vi "Save File Create Default Configuration File.vi"(6 "delimiter (\\t)":string=",", 7 "Default File Create":T1, 8 "Error In":errorcluster={"status"=TRUE, "code"=1172, "source"="Invoke Node System.Reflection.TargetInvocationException: Exception has been thrown by the target of an invocation.\n\tInner Exception: System.ArgumentOutOfRangeException: Index was out of range. Must be non-negative and less than the size of the collection.\r\nParameter name: index <append><b>System.ArgumentOutOfRangeException</b> in GEA2_Toolkit.lvlib:GEA2 Initialize.vi->UTILITY Read Config File.vi->UTILITY Startup and Initialize.vi->HEWH RLT PRAT.vi"}, 11 "File Path In":path=path "C:/Work/Newfi Configuration_StationA.ini") -> (0 "Error Out":errorcluster={"status"=TRUE, "code"=1172, "source"="Invoke Node System.Reflection.TargetInvocationException: Exception has been thrown by the target of an invocation.\n\tInner Exception: System.ArgumentOutOfRangeException: Index was out of range. Must be non-negative and less than the size of the collection.\r\nParameter name: index <append><b>System.ArgumentOutOfRangeException</b> in GEA2_Toolkit.lvlib:GEA2 Initialize.vi->UTILITY Read Config File.vi->UTILITY Startup and Initialize.vi->HEWH RLT PRAT.vi"}, 3 "File Path Out":path=path "C:/Work/Newfi Configuration_StationA_StationD.ini")   [LabVIEW 2020]
uses:
  Type Definitions/UTILITY Default File Create.ctl
  <vilib>/Utility/file.llb/Write Delimited Spreadsheet (string).vi
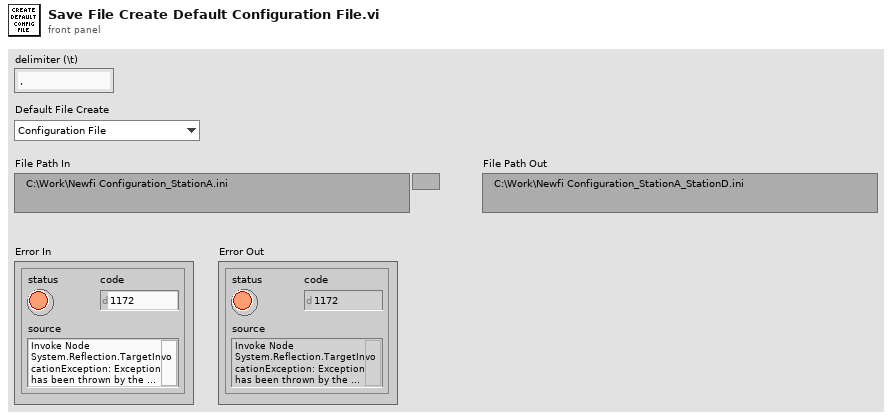
[diagram p1: front panel]
types:
  T1 = typedef "UTILITY Default File Create.ctl" = enum16{"Configuration File", "Debug Search File", "WILT Water Injection Times", "WILT Agilent Assignment", "WILT Save Status Path", "WILT General Config"}
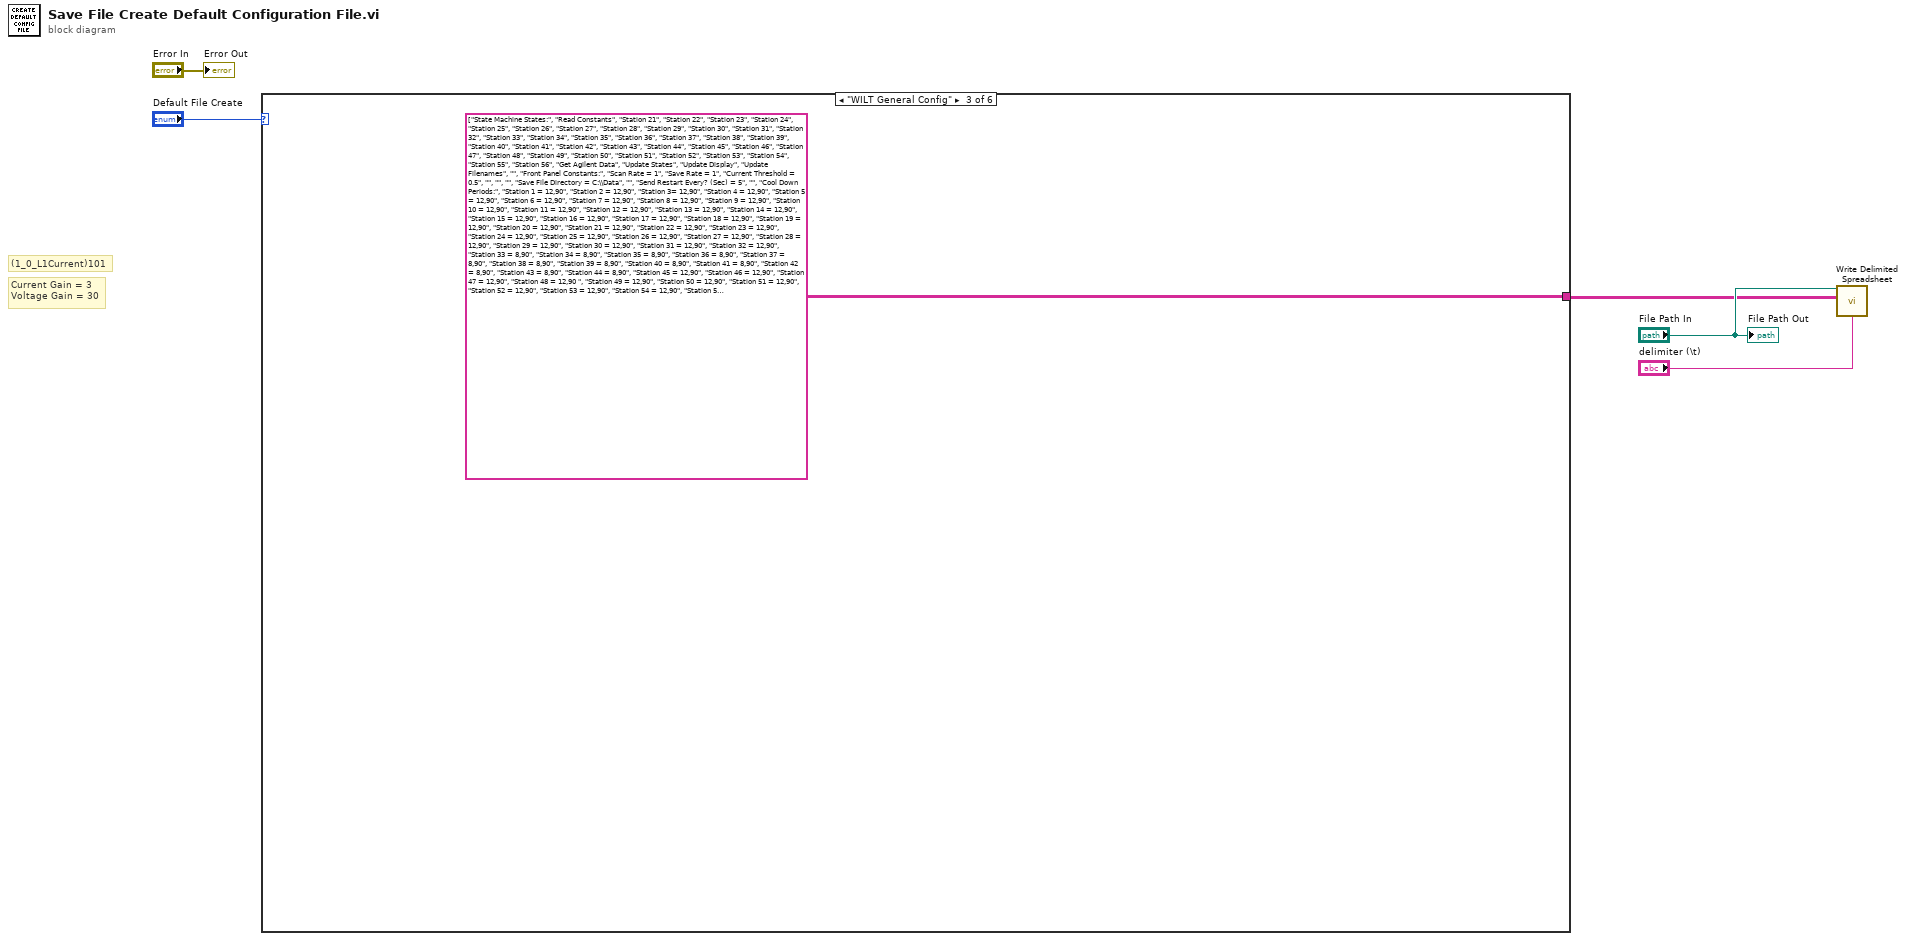
[diagram p0: block diagram]
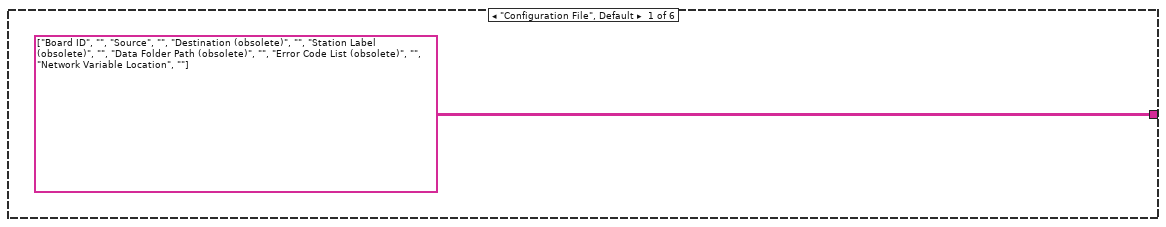
[diagram p2: hidden frame]
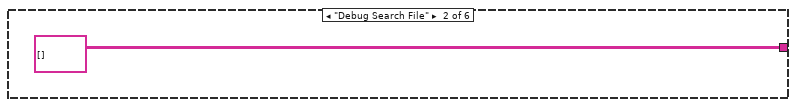
[diagram p3: hidden frame]
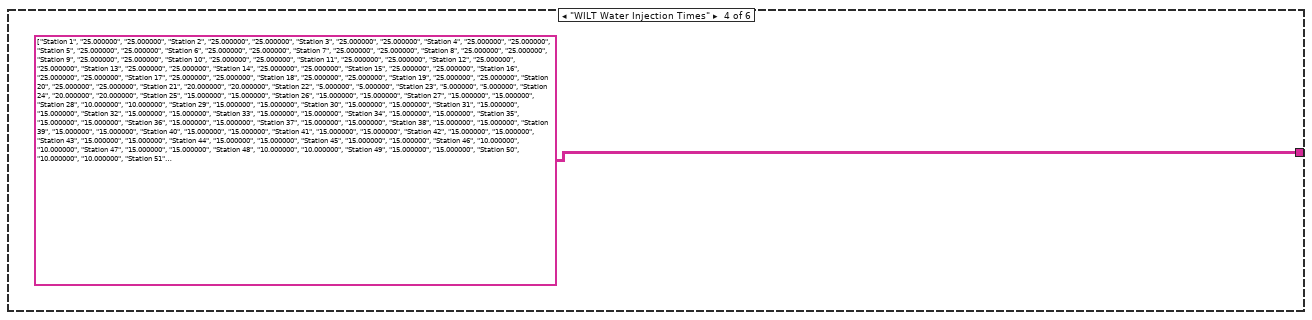
[diagram p4: hidden frame]
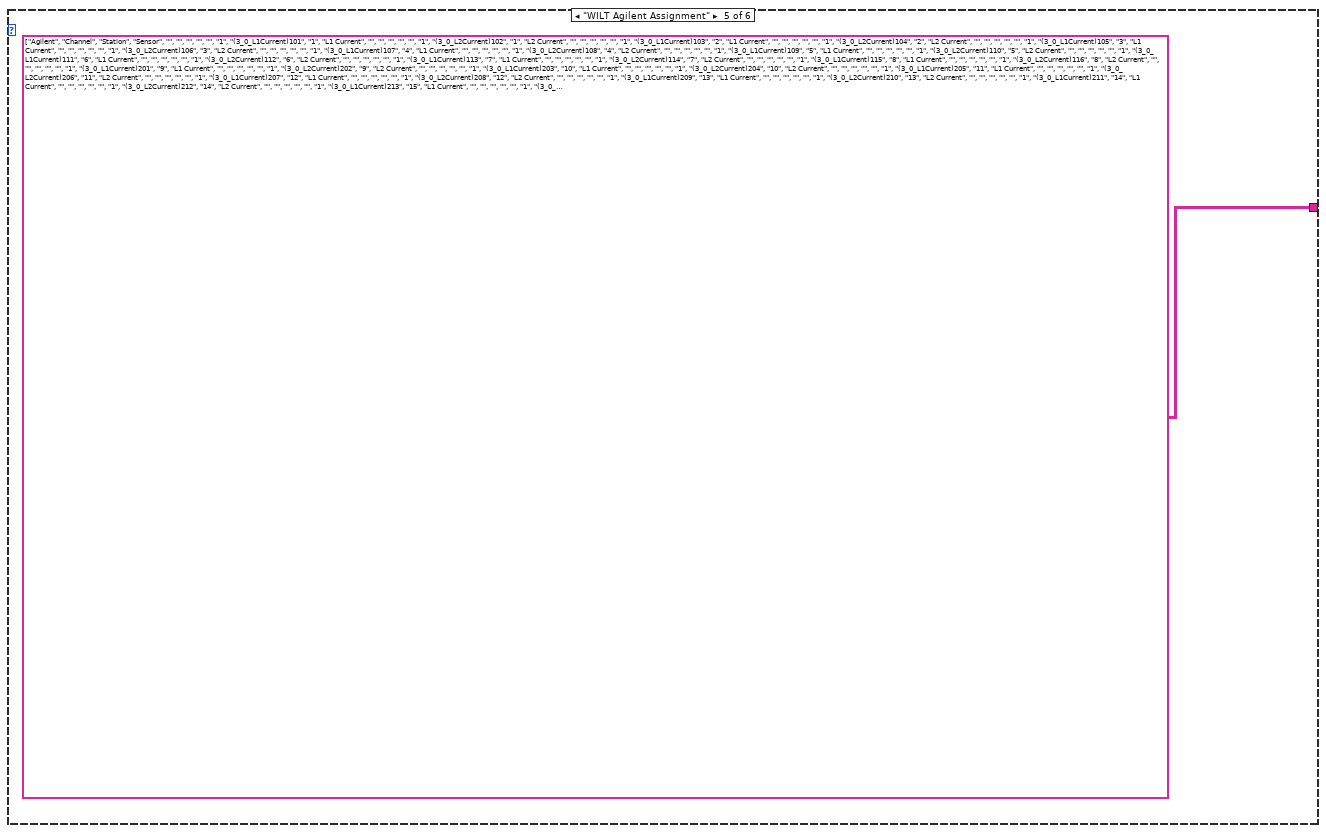
[diagram p5: hidden frame]
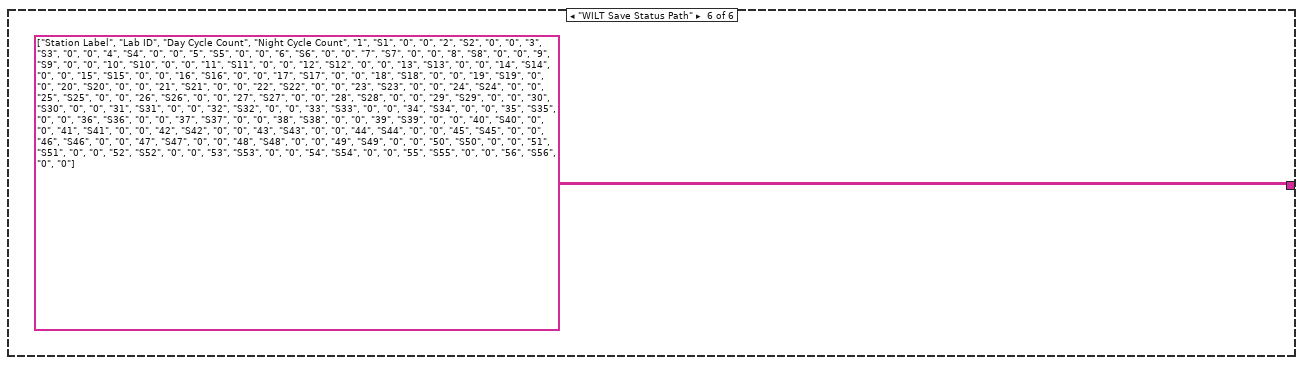
[diagram p6: hidden frame]
diagram:
  # "Current Gain = 3\nVoltage Gain = 30"
  # "(1_0_L1Current)101"
  n1 = case shown="\"WILT General Config\"" "Default File Create" {
    tunnel: [string[][] [["Board ID", ""], ["Source", ""], ["Destination (obsolete)", ""], ["Station Label (obsolete)", ""], ["Data Folder Path (obsolete)", ""], ["Error Code List (obsolete)", ""], ["Network Variable Location", ""]] string[][] [] string[][] [["State Machine States:"], ["Read Constants"], ["Station 21"], ["Station 22"], ["Station 23"], ["Station 24"], ["Station 25"], ["Station 26"], ["Station 27"], ["Station 28"], ["Station 29"], ["Station 30"], ["Station 31"], ["Station 32"], ["Station 33"], ["Station 34"], ["Station 35"], ["Station 36"], ["Station 37"], ["Station 38"], ["Station 39"], ["Station 40"], ["Station 41"], ["Station 42"], ["Station 43"], ["Station 44"], ["Station 45"], ["Station 46"], ["Station 47"], ["Station 48"], ["Station 49"], ["Station 50"], ["Station 51"], ["Station 52"], ["Station 53"], ["Station 54"], ["Station 55"], ["Station 56"], ["Get Agilent Data"], ["Update States"], ["Update Display"], ["Update Filenames"], [""], ["Front Panel Constants:"], ["Scan Rate = 1"], ["Save Rate = 1"], ["Current Threshold = 0.5"], [""], [""], [""], ["Save File Directory = C:\\Data"], [""], ["Send Restart Every? (Sec) = 5"], [""], ["Cool Down Periods:"], ["Station 1 = 12,90"], ["Station 2 = 12,90"], ["Station 3= 12,90"], ["Station 4 = 12,90"], ["Station 5 = 12,90"], ["Station 6 = 12,90"], ["Station 7 = 12,90"], ["Station 8 = 12,90"], ["Station 9 = 12,90"], ["Station 10 = 12,90"], ["Station 11 = 12,90"], ["Station 12 = 12,90"], ["Station 13 = 12,90"], ["Station 14 = 12,90"], ["Station 15 = 12,90"], ["Station 16 = 12,90"], ["Station 17 = 12,90"], ["Station 18 = 12,90"], ["Station 19 = 12,90"], ["Station 20 = 12,90"], ["Station 21 = 12,90"], ["Station 22 = 12,90"], ["Station 23 = 12,90"], ["Station 24 = 12,90"], ["Station 25 = 12,90"], ["Station 26 = 12,90"], ["Station 27 = 12,90"], ["Station 28 = 12,90"], ["Station 29 = 12,90"], ["Station 30 = 12,90"], ["Station 31 = 12,90"], ["Station 32 = 12,90"], ["Station 33 = 8,90"], ["Station 34 = 8,90"], ["Station 35 = 8,90"], ["Station 36 = 8,90"], ["Station 37 = 8,90"], ["Station 38 = 8,90"], ["Station 39 = 8,90"], ["Station 40 = 8,90"], ["Station 41 = 8,90"], ["Station 42 = 8,90"], ["Station 43 = 8,90"], ["Station 44 = 8,90"], ["Station 45 = 12,90"], ["Station 46 = 12,90"], ["Station 47 = 12,90"], ["Station 48 = 12,90 "], ["Station 49 = 12,90"], ["Station 50 = 12,90"], ["Station 51 = 12,90"], ["Station 52 = 12,90"], ["Station 53 = 12,90"], ["Station 54 = 12,90"], ["Station 55 = 12,90"], ["Station 56 = 12,90"]] ("Array") string[][] [["Station 1", "25.000000", "25.000000"], ["Station 2", "25.000000", "25.000000"], ["Station 3", "25.000000", "25.000000"], ["Station 4", "25.000000", "25.000000"], ["Station 5", "25.000000", "25.000000"], ["Station 6", "25.000000", "25.000000"], ["Station 7", "25.000000", "25.000000"], ["Station 8", "25.000000", "25.000000"], ["Station 9", "25.000000", "25.000000"], ["Station 10", "25.000000", "25.000000"], ["Station 11", "25.000000", "25.000000"], ["Station 12", "25.000000", "25.000000"], ["Station 13", "25.000000", "25.000000"], ["Station 14", "25.000000", "25.000000"], ["Station 15", "25.000000", "25.000000"], ["Station 16", "25.000000", "25.000000"], ["Station 17", "25.000000", "25.000000"], ["Station 18", "25.000000", "25.000000"], ["Station 19", "25.000000", "25.000000"], ["Station 20", "25.000000", "25.000000"], ["Station 21", "20.000000", "20.000000"], ["Station 22", "5.000000", "5.000000"], ["Station 23", "5.000000", "5.000000"], ["Station 24", "20.000000", "20.000000"], ["Station 25", "15.000000", "15.000000"], ["Station 26", "15.000000", "15.000000"], ["Station 27", "15.000000", "15.000000"], ["Station 28", "10.000000", "10.000000"], ["Station 29", "15.000000", "15.000000"], ["Station 30", "15.000000", "15.000000"], ["Station 31", "15.000000", "15.000000"], ["Station 32", "15.000000", "15.000000"], ["Station 33", "15.000000", "15.000000"], ["Station 34", "15.000000", "15.000000"], ["Station 35", "15.000000", "15.000000"], ["Station 36", "15.000000", "15.000000"], ["Station 37", "15.000000", "15.000000"], ["Station 38", "15.000000", "15.000000"], ["Station 39", "15.000000", "15.000000"], ["Station 40", "15.000000", "15.000000"], ["Station 41", "15.000000", "15.000000"], ["Station 42", "15.000000", "15.000000"], ["Station 43", "15.000000", "15.000000"], ["Station 44", "15.000000", "15.000000"], ["Station 45", "15.000000", "15.000000"], ["Station 46", "10.000000", "10.000000"], ["Station 47", "15.000000", "15.000000"], ["Station 48", "10.000000", "10.000000"], ["Station 49", "15.000000", "15.000000"], ["Station 50", "10.000000", "10.000000"], ["Station 51", "15.000000", "15.000000"], ["Station 52", "15.000000", "15.000000"], ["Station 53", "15.000000", "15.000000"], ["Station 54", "15.000000", "15.000000"], ["Station 55", "15.000000", "15.000000"], ["Station 56", "15.000000", "15.000000"]] ("Array") string[][] [["Agilent", "Channel", "Station", "Sensor", "", "", "", "", ""], ["1", "(3_0_L1Current)101", "1", "L1 Current", "", "", "", "", ""], ["1", "(3_0_L2Current)102", "1", "L2 Current", "", "", "", "", ""], ["1", "(3_0_L1Current)103", "2", "L1 Current", "", "", "", "", ""], ["1", "(3_0_L2Current)104", "2", "L2 Current", "", "", "", "", ""], ["1", "(3_0_L1Current)105", "3", "L1 Current", "", "", "", "", ""], ["1", "(3_0_L2Current)106", "3", "L2 Current", "", "", "", "", ""], ["1", "(3_0_L1Current)107", "4", "L1 Current", "", "", "", "", ""], ["1", "(3_0_L2Current)108", "4", "L2 Current", "", "", "", "", ""], ["1", "(3_0_L1Current)109", "5", "L1 Current", "", "", "", "", ""], ["1", "(3_0_L2Current)110", "5", "L2 Current", "", "", "", "", ""], ["1", "(3_0_L1Current)111", "6", "L1 Current", "", "", "", "", ""], ["1", "(3_0_L2Current)112", "6", "L2 Current", "", "", "", "", ""], ["1", "(3_0_L1Current)113", "7", "L1 Current", "", "", "", "", ""], ["1", "(3_0_L2Current)114", "7", "L2 Current", "", "", "", "", ""], ["1", "(3_0_L1Current)115", "8", "L1 Current", "", "", "", "", ""], ["1", "(3_0_L2Current)116", "8", "L2 Current", "", "", "", "", ""], ["1", "(3_0_L1Current)201", "9", "L1 Current", "", "", "", "", ""], ["1", "(3_0_L2Current)202", "9", "L2 Current", "", "", "", "", ""], ["1", "(3_0_L1Current)203", "10", "L1 Current", "", "", "", "", ""], ["1", "(3_0_L2Current)204", "10", "L2 Current", "", "", "", "", ""], ["1", "(3_0_L1Current)205", "11", "L1 Current", "", "", "", "", ""], ["1", "(3_0_L2Current)206", "11", "L2 Current", "", "", "", "", ""], ["1", "(3_0_L1Current)207", "12", "L1 Current", "", "", "", "", ""], ["1", "(3_0_L2Current)208", "12", "L2 Current", "", "", "", "", ""], ["1", "(3_0_L1Current)209", "13", "L1 Current", "", "", "", "", ""], ["1", "(3_0_L2Current)210", "13", "L2 Current", "", "", "", "", ""], ["1", "(3_0_L1Current)211", "14", "L1 Current", "", "", "", "", ""], ["1", "(3_0_L2Current)212", "14", "L2 Current", "", "", "", "", ""], ["1", "(3_0_L1Current)213", "15", "L1 Current", "", "", "", "", ""], ["1", "(3_0_L2Current)214", "15", "L2 Current", "", "", "", "", ""], ["1", "(3_0_L1Current)215", "16", "L1 Current", "", "", "", "", ""], ["1", "(3_0_L2Current)216", "16", "L2 Current", "", "", "", "", ""], ["1", "(3_0_L1Current)301", "17", "L1 Current", "", "", "", "", ""], ["1", "(3_0_L2Current)302", "17", "L2 Current", "", "", "", "", ""], ["1", "(3_0_L1Current)303", "18", "L1 Current", "", "", "", "", ""], ["1", "(3_0_L2Current)304", "18", "L2 Current", "", "", "", "", ""], ["1", "(3_0_L1Current)305", "19", "L1 Current", "", "", "", "", ""], ["1", "(3_0_L2Current)306", "19", "L2 Current", "", "", "", "", ""], ["1", "(3_0_L1Current)307", "20", "L1 Current", "", "", "", "", ""], ["1", "(3_0_L2Current)308", "20", "L2 Current", "", "", "", "", ""], ["1", "(3_0_L1Current)309", "21", "L1 Current", "", "", "", "", ""], ["1", "(3_0_L2Current)310", "21", "L2 Current", "", "", "", "", ""], ["1", "(3_0_L1Current)311", "22", "L1 Current", "", "", "", "", ""], ["1", "(3_0_L2Current)312", "22", "L2 Current", "", "", "", "", ""], ["1", "(3_0_L1Current)313", "23", "L1 Current", "", "", "", "", ""], ["1", "(3_0_L2Current)314", "23", "L2 Current", "", "", "", "", ""], ["1", "(3_0_L1Current)315", "24", "L1 Current", "", "", "", "", ""], ["1", "(3_0_L2Current)316", "24", "L2 Current", "", "", "", "", ""], ["2", "(3_0_L1Current)101", "25", "L1 Current", "", "", "", "", ""], ["2", "(3_0_L2Current)102", "25", "L2 Current", "", "", "", "", ""], ["2", "(3_0_L1Current)103", "26", "L1 Current", "", "", "", "", ""], ["2", "(3_0_L2Current)104", "26", "L2 Current", "", "", "", "", ""], ["2", "(3_0_L1Current)105", "27", "L1 Current", "", "", "", "", ""], ["2", "(3_0_L2Current)106", "27", "L2 Current", "", "", "", "", ""], ["2", "(3_0_L1Current)107", "28", "L1 Current", "", "", "", "", ""], ["2", "(3_0_L2Current)108", "28", "L2 Current", "", "", "", "", ""], ["2", "(3_0_L1Current)109", "29", "L1 Current", "", "", "", "", ""], ["2", "(3_0_L2Current)110", "29", "L2 Current", "", "", "", "", ""], ["2", "(3_0_L1Current)111", "30", "L1 Current", "", "", "", "", ""], ["2", "(3_0_L2Current)112", "30", "L2 Current", "", "", "", "", ""], ["2", "(3_0_L1Current)113", "31", "L1 Current", "", "", "", "", ""], ["2", "(3_0_L2Current)114", "31", "L2 Current", "", "", "", "", ""], ["2", "(3_0_L1Current)115", "32", "L1 Current", "", "", "", "", ""], ["2", "(3_0_L2Current)116", "32", "L2 Current", "", "", "", "", ""], ["2", "(30_0_Volts)201", "5", "Volts", "", "", "", "", ""], ["2", "(30_0_Volts)202", "6", "Volts", "", "", "", "", ""], ["2", "(30_0_Volts)203", "7", "Volts", "", "", "", "", ""], ["2", "(30_0_Volts)204", "8", "Volts", "", "", "", "", ""], ["2", "(30_0_Volts)205", "9", "Volts", "", "", "", "", ""], ["2", "(30_0_Volts)206", "10", "Volts", "", "", "", "", ""], ["2", "(30_0_Volts)207", "11", "Volts", "", "", "", "", ""], ["2", "(30_0_Volts)208", "12", "Volts", "", "", "", "", ""], ["2", "(30_0_Volts)209", "13", "Volts", "", "", "", "", ""], ["2", "(30_0_Volts)210", "14", "Volts", "", "", "", "", ""], ["2", "(30_0_Volts)211", "21", "Volts", "", "", "", "", ""], ["2", "(30_0_Volts)211", "22", "Volts", "", "", "", "", ""], ["2", "(30_0_Volts)211", "23", "Volts", "", "", "", "", ""], ["2", "(30_0_Volts)212", "24", "Volts", "", "", "", "", ""], ["2", "(30_0_Volts)212", "25", "Volts", "", "", "", "", ""], ["2", "(30_0_Volts)212", "26", "Volts", "", "", "", "", ""], ["2", "(30_0_Volts)213", "27", "Volts", "", "", "", "", ""], ["2", "(30_0_Volts)213", "28", "Volts", "", "", "", "", ""], ["2", "(30_0_Volts)213", "29", "Volts", "", "", "", "", ""], ["2", "(30_0_Volts)214", "30", "Volts", "", "", "", "", ""], ["2", "(30_0_Volts)214", "31", "Volts", "", "", "", "", ""], ["2", "(30_0_Volts)214", "32", "Volts", "", "", "", "", ""], ["2", "(30_0_Volts)215", "15", "Volts", "", "", "", "", ""], ["2", "(30_0_Volts)216", "16", "Volts", "", "", "", "", ""], ["2", "301", "1", "Water Valve", "", "", "", "", ""], ["2", "302", "2", "Water Valve", "", "", "", "", ""], ["2", "303", "3", "Water Valve", "", "", "", "", ""], ["2", "304", "4", "Water Valve", "", "", "", "", ""], ["2", "305", "5", "Water Valve", "", "", "", "", ""], ["2", "306", "6", "Water Valve", "", "", "", "", ""], ["2", "307", "7", "Water Valve", "", "", "", "", ""], ["2", "308", "8", "Water Valve", "", "", "", "", ""], ["2", "309", "9", "Water Valve", "", "", "", "", ""], ["2", "310", "10", "Water Valve", "", "", "", "", ""], ["2", "311", "11", "Water Valve", "", "", "", "", ""], ["2", "312", "12", "Water Valve", "", "", "", "", ""], ["2", "313", "13", "Water Valve", "", "", "", "", ""], ["2", "314", "14", "Water Valve", "", "", "", "", ""], ["2", "315", "15", "Water Valve", "", "", "", "", ""], ["2", "316", "16", "Water Valve", "", "", "", "", ""], ["2", "317", "17", "Water Valve", "", "", "", "", ""], ["2", "318", "18", "Water Valve", "", "", "", "", ""], ["2", "319", "19", "Water Valve", "", "", "", "", ""], ["2", "320", "20", "Water Valve", "", "", "", "", ""], ["3", "101", "21", "Water Valve", "", "", "", "", ""], ["3", "102", "22", "Water Valve", "", "", "", "", ""], ["3", "103", "23", "Water Valve", "", "", "", "", ""], ["3", "104", "24", "Water Valve", "", "", "", "", ""], ["3", "105", "25", "Water Valve", "", "", "", "", ""], ["3", "106", "26", "Water Valve", "", "", "", "", ""], ["3", "107", "27", "Water Valve", "", "", "", "", ""], ["3", "108", "28", "Water Valve", "", "", "", "", ""], ["3", "109", "29", "Water Valve", "", "", "", "", ""], ["3", "110", "30", "Water Valve", "", "", "", "", ""], ["3", "111", "31", "Water Valve", "", "", "", "", ""], ["3", "112", "32", "Water Valve", "", "", "", "", ""], ["3", "113", "", "", "", "", "", "", ""], ["3", "114", "", "", "", "", "", "", ""], ["3", "115", "", "", "", "", "", "", ""], ["3", "116", "", "", "", "", "", "", ""], ["3", "117", "", "", "", "", "", "", ""], ["3", "118", "", "", "", "", "", "", ""], ["3", "119", "", "", "", "", "", "", ""], ["3", "120", "", "", "", "", "", "", ""], ["3", "201", "1", "Temperature", "", "", "", "", ""], ["3", "202", "2", "Temperature", "", "", "", "", ""], ["3", "203", "3", "Temperature", "", "", "", "", ""], ["3", "204", "4", "Temperature", "", "", "", "", ""], ["3", "205", "5", "Temperature", "", "", "", "", ""], ["3", "206", "6", "Temperature", "", "", "", "", ""], ["3", "207", "7", "Temperature", "", "", "", "", ""], ["3", "208", "8", "Temperature", "", "", "", "", ""], ["3", "209", "9", "Temperature", "", "", "", "", ""], ["3", "210", "10", "Temperature", "", "", "", "", ""], ["3", "211", "11", "Temperature", "", "", "", "", ""], ["3", "212", "12", "Temperature", "", "", "", "", ""], ["3", "213", "13", "Temperature", "", "", "", "", ""], ["3", "214", "14", "Temperature", "", "", "", "", ""], ["3", "215", "15", "Temperature", "", "", "", "", ""], ["3", "216", "16", "Temperature", "", "", "", "", ""], ["3", "217", "17", "Temperature", "", "", "", "", ""], ["3", "218", "18", "Temperature", "", "", "", "", ""], ["3", "219", "19", "Temperature", "", "", "", "", ""], ["3", "220", "20", "Temperature", "", "", "", "", ""], ["3", "301", "21", "Temperature", "", "", "", "", ""], ["3", "302", "22", "Temperature", "", "", "", "", ""], ["3", "303", "23", "Temperature", "", "", "", "", ""], ["3", "304", "24", "Temperature", "", "", "", "", ""], ["3", "305", "25", "Temperature", "", "", "", "", ""], ["3", "306", "26", "Temperature", "", "", "", "", ""], ["3", "307", "27", "Temperature", "", "", "", "", ""], ["3", "308", "28", "Temperature", "", "", "", "", ""], ["3", "309", "29", "Temperature", "", "", "", "", ""], ["3", "310", "30", "Temperature", "", "", "", "", ""], ["3", "311", "31", "Temperature", "", "", "", "", ""], ["3", "312", "32", "Temperature", "", "", "", "", ""], ["3", "(30_0_Volts)313", "1", "Volts", "", "", "", "", ""], ["3", "(30_0_Volts)314", "2", "Volts", "", "", "", "", ""], ["3", "(30_0_Volts)315", "3", "Volts", "", "", "", "", ""], ["3", "(30_0_Volts)316", "4", "Volts", "", "", "", "", ""], ["4", "(3_0_L1Current)101", "33", "L1 Current", "", "", "", "", ""], ["4", "(3_0_L2Current)102", "33", "L2 Current", "", "", "", "", ""], ["4", "(3_0_L1Current)103", "34", "L1 Current", "", "", "", "", ""], ["4", "(3_0_L2Current)104", "34", "L2 Current", "", "", "", "", ""], ["4", "(3_0_L1Current)105", "35", "L1 Current", "", "", "", "", ""], ["4", "(3_0_L2Current)106", "35", "L2 Current", "", "", "", "", ""], ["4", "(3_0_L1Current)107", "36", "L1 Current", "", "", "", "", ""], ["4", "(3_0_L2Current)108", "36", "L2 Current", "", "", "", "", ""], ["4", "(3_0_L1Current)109", "37", "L1 Current", "", "", "", "", ""], ["4", "(3_0_L2Current)110", "37", "L2 Current", "", "", "", "", ""], ["4", "(3_0_L1Current)111", "38", "L1 Current", "", "", "", "", ""], ["4", "(3_0_L2Current)112", "38", "L2 Current", "", "", "", "", ""], ["4", "(3_0_L1Current)113", "39", "L1 Current", "", "", "", "", ""], ["4", "(3_0_L2Current)114", "39", "L2 Current", "", "", "", "", ""], ["4", "(3_0_L1Current)115", "40", "L1 Current", "", "", "", "", ""], ["4", "(3_0_L2Current)116", "40", "L2 Current", "", "", "", "", ""], ["4", "(3_0_L1Current)201", "41", "L1 Current", "", "", "", "", ""], ["4", "(3_0_L2Current)202", "41", "L2 Current", "", "", "", "", ""], ["4", "(3_0_L1Current)203", "42", "L1 Current", "", "", "", "", ""], ["4", "(3_0_L2Current)204", "42", "L2 Current", "", "", "", "", ""], ["4", "(3_0_L1Current)205", "43", "L1 Current", "", "", "", "", ""], ["4", "(3_0_L2Current)206", "43", "L2 Current", "", "", "", "", ""], ["4", "(3_0_L1Current)207", "44", "L1 Current", "", "", "", "", ""], ["4", "(3_0_L2Current)208", "44", "L2 Current", "", "", "", "", ""], ["4", "(3_0_L1Current)209", "45", "L1 Current", "", "", "", "", ""], ["4", "(3_0_L2Current)210", "45", "L2 Current", "", "", "", "", ""], ["4", "(3_0_L1Current)211", "46", "L1 Current", "", "", "", "", ""], ["4", "(3_0_L2Current)212", "46", "L2 Current", "", "", "", "", ""], ["4", "(3_0_L1Current)213", "47", "L1 Current", "", "", "", "", ""], ["4", "(3_0_L2Current)214", "47", "L2 Current", "", "", "", "", ""], ["4", "(3_0_L1Current)215", "48", "L1 Current", "", "", "", "", ""], ["4", "(3_0_L2Current)216", "48", "L2 Current", "", "", "", "", ""], ["4", "(3_0_L1Current)301", "49", "L1 Current", "", "", "", "", ""], ["4", "(3_0_L2Current)302", "49", "L2 Current", "", "", "", "", ""], ["4", "(3_0_L1Current)303", "50", "L1 Current", "", "", "", "", ""], ["4", "(3_0_L2Current)304", "50", "L2 Current", "", "", "", "", ""], ["4", "(3_0_L1Current)305", "51", "L1 Current", "", "", "", "", ""], ["4", "(3_0_L2Current)306", "51", "L2 Current", "", "", "", "", ""], ["4", "(3_0_L1Current)307", "52", "L1 Current", "", "", "", "", ""], ["4", "(3_0_L2Current)308", "52", "L2 Current", "", "", "", "", ""], ["4", "(3_0_L1Current)309", "53", "L1 Current", "", "", "", "", ""], ["4", "(3_0_L2Current)310", "53", "L2 Current", "", "", "", "", ""], ["4", "(3_0_L1Current)311", "54", "L1 Current", "", "", "", "", ""], ["4", "(3_0_L2Current)312", "54", "L2 Current", "", "", "", "", ""], ["4", "(3_0_L1Current)313", "55", "L1 Current", "", "", "", "", ""], ["4", "(3_0_L2Current)314", "55", "L2 Current", "", "", "", "", ""], ["4", "(3_0_L1Current)315", "56", "L1 Current", "", "", "", "", ""], ["4", "(3_0_L2Current)316", "56", "L2 Current", "", "", "", "", ""], ["5", "101", "33", "Water Valve", "", "", "", "", ""], ["5", "102", "34", "Water Valve", "", "", "", "", ""], ["5", "103", "35", "Water Valve", "", "", "", "", ""], ["5", "104", "36", "Water Valve", "", "", "", "", ""], ["5", "105", "37", "Water Valve", "", "", "", "", ""], ["5", "106", "38", "Water Valve", "", "", "", "", ""], ["5", "107", "39", "Water Valve", "", "", "", "", ""], ["5", "108", "40", "Water Valve", "", "", "", "", ""], ["5", "109", "41", "Water Valve", "", "", "", "", ""], ["5", "110", "42", "Water Valve", "", "", "", "", ""], ["5", "111", "43", "Water Valve", "", "", "", "", ""], ["5", "112", "44", "Water Valve", "", "", "", "", ""], ["5", "113", "45", "Water Valve", "", "", "", "", ""], ["5", "114", "46", "Water Valve", "", "", "", "", ""], ["5", "115", "47", "Water Valve", "", "", "", "", ""], ["5", "116", "48", "Water Valve", "", "", "", "", ""], ["5", "117", "49", "Water Valve", "", "", "", "", ""], ["5", "118", "50", "Water Valve", "", "", "", "", ""], ["5", "119", "51", "Water Valve", "", "", "", "", ""], ["5", "120", "52", "Water Valve", "", "", "", "", ""], ["5", "201", "53", "Water Valve", "", "", "", "", ""], ["5", "202", "54", "Water Valve", "", "", "", "", ""], ["5", "203", "55", "Water Valve", "", "", "", "", ""], ["5", "204", "56", "Water Valve", "", "", "", "", ""], ["5", "205", "", "", "", "", "", "", ""], ["5", "206", "", "", "", "", "", "", ""], ["5", "207", "", "", "", "", "", "", ""], ["5", "208", "", "", "", "", "", "", ""], ["5", "209", "", "", "", "", "", "", ""], ["5", "210", "", "", "", "", "", "", ""], ["5", "211", "", "", "", "", "", "", ""], ["5", "212", "", "", "", "", "", "", ""], ["5", "213", "", "", "", "", "", "", ""], ["5", "214", "", "", "", "", "", "", ""], ["5", "215", "", "", "", "", "", "", ""], ["5", "216", "", "", "", "", "", "", ""], ["5", "217", "", "", "", "", "", "", ""], ["5", "218", "", "", "", "", "", "", ""], ["5", "219", "", "", "", "", "", "", ""], ["5", "220", "", "", "", "", "", "", ""], ["5", "301", "21", "Start Button", "", "", "", "", ""], ["5", "302", "22", "Start Button", "", "", "", "", ""], ["5", "303", "23", "Start Button", "", "", "", "", ""], ["5", "304", "24", "Start Button", "", "", "", "", ""], ["5", "305", "25", "Start Button", "", "", "", "", ""], ["5", "306", "26", "Start Button", "", "", "", "", ""], ["5", "307", "27", "Start Button", "", "", "", "", ""], ["5", "308", "28", "Start Button", "", "", "", "", ""], ["5", "309", "29", "Start Button", "", "", "", "", ""], ["5", "310", "30", "Start Button", "", "", "", "", ""], ["5", "311", "31", "Start Button", "", "", "", "", ""], ["5", "312", "32", "Start Button", "", "", "", "", ""], ["5", "313", "", "", "", "", "", "", ""], ["5", "314", "", "", "", "", "", "", ""], ["5", "315", "", "", "", "", "", "", ""], ["5", "316", "", "", "", "", "", "", ""], ["5", "317", "", "", "", "", "", "", ""], ["5", "318", "", "", "", "", "", "", ""], ["5", "319", "", "", "", "", "", "", ""], ["5", "320", "", "", "", "", "", "", ""], ["6", "101", "33", "Temperature", "", "", "", "", ""], ["6", "102", "34", "Temperature", "", "", "", "", ""], ["6", "103", "35", "Temperature", "", "", "", "", ""], ["6", "104", "36", "Temperature", "", "", "", "", ""], ["6", "105", "37", "Temperature", "", "", "", "", ""], ["6", "106", "38", "Temperature", "", "", "", "", ""], ["6", "107", "39", "Temperature", "", "", "", "", ""], ["6", "108", "40", "Temperature", "", "", "", "", ""], ["6", "109", "41", "Temperature", "", "", "", "", ""], ["6", "110", "42", "Temperature", "", "", "", "", ""], ["6", "111", "43", "Temperature", "", "", "", "", ""], ["6", "112", "44", "Temperature", "", "", "", "", ""], ["6", "113", "45", "Temperature", "", "", "", "", ""], ["6", "114", "46", "Temperature", "", "", "", "", ""], ["6", "115", "47", "Temperature", "", "", "", "", ""], ["6", "116", "48", "Temperature", "", "", "", "", ""], ["6", "117", "49", "Temperature", "", "", "", "", ""], ["6", "118", "50", "Temperature", "", "", "", "", ""], ["6", "119", "51", "Temperature", "", "", "", "", ""], ["6", "120", "52", "Temperature", "", "", "", "", ""], ["6", "201", "53", "Temperature", "", "", "", "", ""], ["6", "202", "54", "Temperature", "", "", "", "", ""], ["6", "203", "55", "Temperature", "", "", "", "", ""], ["6", "204", "56", "Temperature", "", "", "", "", ""], ["6", "(30_0_Volts)205", "33", "Volts", "", "", "", "", ""], ["6", "(30_0_Volts)205", "34", "Volts", "", "", "", "", ""], ["6", "(30_0_Volts)205", "35", "Volts", "", "", "", "", ""], ["6", "(30_0_Volts)206", "36", "Volts", "", "", "", "", ""], ["6", "(30_0_Volts)206", "37", "Volts", "", "", "", "", ""], ["6", "(30_0_Volts)206", "38", "Volts", "", "", "", "", ""], ["6", "(30_0_Volts)207", "39", "Volts", "", "", "", "", ""], ["6", "(30_0_Volts)207", "40", "Volts", "", "", "", "", ""], ["6", "(30_0_Volts)208", "42", "Volts", "", "", "", "", ""], ["6", "(30_0_Volts)208", "43", "Volts", "", "", "", "", ""], ["6", "(30_0_Volts)208", "44", "Volts", "", "", "", "", ""], ["6", "(30_0_Volts)209", "45", "Volts", "", "", "", "", ""], ["6", "(30_0_Volts)209", "46", "Volts", "", "", "", "", ""], ["6", "(30_0_Volts)209", "47", "Volts", "", "", "", "", ""], ["6", "(30_0_Volts)210", "45", "Volts (208)", "", "", "", "", ""], ["6", "211", "45", "SW (208)", "", "", "", "", ""], ["6", "(30_0_Volts)212", "48", "Volts", "", "", "", "", ""], ["6", "(30_0_Volts)212", "49", "Volts", "", "", "", "", ""], ["6", "(30_0_Volts)212", "50", "Volts", "", "", "", "", ""], ["6", "213", "48", "SW (208)", "", "", "", "", ""], ["6", "(30_0_Volts)214", "51", "Volts (208)", "", "", "", "", ""], ["6", "215", "51", "SW (208)", "", "", "", "", ""], ["6", "(30_0_Volts)216", "54", "Volts", "", "", "", "", ""], ["6", "(30_0_Volts)216", "55", "Volts", "", "", "", "", ""], ["6", "(30_0_Volts)216", "56", "Volts", "", "", "", "", ""], ["6", "(30_0_Volts)301", "17", "Volts", "", "", "", "", ""], ["6", "(30_0_Volts)302", "18", "Volts", "", "", "", "", ""], ["6", "(30_0_Volts)303", "19", "Volts", "", "", "", "", ""], ["6", "(30_0_Volts)304", "20", "Volts", "", "", "", "", ""], ["6", "(30_0_Volts)305", "51", "Volts", "", "", "", "", ""], ["6", "(30_0_Volts)305", "52", "Volts", "", "", "", "", ""], ["6", "(30_0_Volts)305", "53", "Volts", "", "", "", "", ""], ["6", "(30_0_Volts)306", "48", "Volts (208)", "", "", "", "", ""], ["6", "307", "", "", "", "", "", "", ""], ["6", "308", "", "", "", "", "", "", ""], ["6", "309", "", "", "", "", "", "", ""], ["6", "310", "", "", "", "", "", "", ""], ["6", "311", "", "", "", "", "", "", ""], ["6", "312", "", "", "", "", "", "", ""], ["6", "313", "", "", "", "", "", "", ""], ["6", "314", "", "", "", "", "", "", ""], ["6", "315", "", "", "", "", "", "", ""], ["6", "316", "", "", "", "", "", "", ""], ["7", "101", "33", "Start Button", "", "", "", "", ""], ["7", "102", "34", "Start Button", "", "", "", "", ""], ["7", "103", "35", "Start Button", "", "", "", "", ""], ["7", "104", "36", "Start Button", "", "", "", "", ""], ["7", "105", "37", "Start Button", "", "", "", "", ""], ["7", "106", "38", "Start Button", "", "", "", "", ""], ["7", "107", "39", "Start Button", "", "", "", "", ""], ["7", "108", "40", "Start Button", "", "", "", "", ""], ["7", "109", "41", "Start Button", "", "", "", "", ""], ["7", "110", "42", "Start Button", "", "", "", "", ""], ["7", "111", "43", "Start Button", "", "", "", "", ""], ["7", "112", "44", "Start Button", "", "", "", "", ""], ["7", "113", "45", "Start Button", "", "", "", "", ""], ["7", "114", "46", "Start Button", "", "", "", "", ""], ["7", "115", "47", "Start Button", "", "", "", "", ""], ["7", "116", "48", "Start Button", "", "", "", "", ""], ["7", "117", "49", "Start Button", "", "", "", "", ""], ["7", "118", "50", "Start Button", "", "", "", "", ""], ["7", "119", "51", "Start Button", "", "", "", "", ""], ["7", "120", "52", "Start Button", "", "", "", "", ""], ["7", "201", "53", "Start Button", "", "", "", "", ""], ["7", "202", "54", "Start Button", "", "", "", "", ""], ["7", "203", "55", "Start Button", "", "", "", "", ""], ["7", "204", "56", "Start Button", "", "", "", "", ""], ["7", "205", "", "", "", "", "", "", ""], ["7", "206", "", "", "", "", "", "", ""], ["7", "207", "", "", "", "", "", "", ""], ["7", "208", "", "", "", "", "", "", ""], ["7", "209", "", "", "", "", "", "", ""], ["7", "210", "", "", "", "", "", "", ""], ["7", "211", "", "", "", "", "", "", ""], ["7", "212", "", "", "", "", "", "", ""], ["7", "213", "", "", "", "", "", "", ""], ["7", "214", "", "", "", "", "", "", ""], ["7", "215", "", "", "", "", "", "", ""], ["7", "216", "", "", "", "", "", "", ""], ["7", "217", "", "", "", "", "", "", ""], ["7", "218", "", "", "", "", "", "", ""], ["7", "219", "", "", "", "", "", "", ""], ["7", "220", "", "", "", "", "", "", ""], ["7", "301", "", "", "", "", "", "", ""], ["7", "302", "", "", "", "", "", "", ""], ["7", "303", "", "", "", "", "", "", ""], ["7", "304", "", "", "", "", "", "", ""], ["7", "305", "", "", "", "", "", "", ""], ["7", "306", "", "", "", "", "", "", ""], ["7", "307", "", "", "", "", "", "", ""], ["7", "308", "", "", "", "", "", "", ""], ["7", "309", "", "", "", "", "", "", ""], ["7", "310", "", "", "", "", "", "", ""], ["7", "311", "", "", "", "", "", "", ""], ["7", "312", "", "", "", "", "", "", ""], ["7", "313", "", "", "", "", "", "", ""], ["7", "314", "", "", "", "", "", "", ""], ["7", "315", "", "", "", "", "", "", ""], ["7", "316", "", "", "", "", "", "", ""], ["7", "317", "", "", "", "", "", "", ""], ["7", "318", "", "", "", "", "", "", ""], ["7", "319", "", "", "", "", "", "", ""], ["7", "320", "", "", "", "", "", "", ""], ["", "", "", "", "", "", "", "", ""]] ("Array") string[][] [["Station Label", "Lab ID", "Day Cycle Count", "Night Cycle Count"], ["1", "S1", "0", "0"], ["2", "S2", "0", "0"], ["3", "S3", "0", "0"], ["4", "S4", "0", "0"], ["5", "S5", "0", "0"], ["6", "S6", "0", "0"], ["7", "S7", "0", "0"], ["8", "S8", "0", "0"], ["9", "S9", "0", "0"], ["10", "S10", "0", "0"], ["11", "S11", "0", "0"], ["12", "S12", "0", "0"], ["13", "S13", "0", "0"], ["14", "S14", "0", "0"], ["15", "S15", "0", "0"], ["16", "S16", "0", "0"], ["17", "S17", "0", "0"], ["18", "S18", "0", "0"], ["19", "S19", "0", "0"], ["20", "S20", "0", "0"], ["21", "S21", "0", "0"], ["22", "S22", "0", "0"], ["23", "S23", "0", "0"], ["24", "S24", "0", "0"], ["25", "S25", "0", "0"], ["26", "S26", "0", "0"], ["27", "S27", "0", "0"], ["28", "S28", "0", "0"], ["29", "S29", "0", "0"], ["30", "S30", "0", "0"], ["31", "S31", "0", "0"], ["32", "S32", "0", "0"], ["33", "S33", "0", "0"], ["34", "S34", "0", "0"], ["35", "S35", "0", "0"], ["36", "S36", "0", "0"], ["37", "S37", "0", "0"], ["38", "S38", "0", "0"], ["39", "S39", "0", "0"], ["40", "S40", "0", "0"], ["41", "S41", "0", "0"], ["42", "S42", "0", "0"], ["43", "S43", "0", "0"], ["44", "S44", "0", "0"], ["45", "S45", "0", "0"], ["46", "S46", "0", "0"], ["47", "S47", "0", "0"], ["48", "S48", "0", "0"], ["49", "S49", "0", "0"], ["50", "S50", "0", "0"], ["51", "S51", "0", "0"], ["52", "S52", "0", "0"], ["53", "S53", "0", "0"], ["54", "S54", "0", "0"], ["55", "S55", "0", "0"], ["56", "S56", "0", "0"]] ("Array")] -> w1
    frame "Configuration File", Default {
    }
    frame "Debug Search File" {
    }
    frame "WILT General Config" {
    }
    frame "WILT Water Injection Times" {
    }
    frame "WILT Agilent Assignment" {
    }
    frame "WILT Save Status Path" {
    }
  }
  n2 = call-poly <vilib>:"Write Delimited Spreadsheet.vi"("file path (dialog if empty)"="File Path In", "2D data"=w1, "delimiter (\\t)"="delimiter (\\t)") -> ()  [unwired: 11 in, 2 out]
  "Error Out" <- "Error In"
  "File Path Out" <- "File Path In"
